vi "4080_display_source.vi"(0 "Module Address":u8) -> ()   [LabVIEW 2010]
panel:
  in  "Port Name":string="MainNetwork"
  in  "Data Source":u16(ring) items=["Counter0", "Counter1", "Host"]
  out "Read":string=">+00.000"
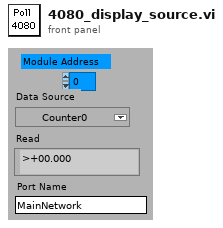
[diagram p1: front panel]
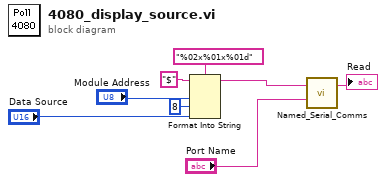
[diagram p0: block diagram]
diagram:
  n1 = Format Into String(format string="%02x%01x%01d", initial string="$", "Module Address", u8 8 ("Channel"), "Data Source") -> (resulting string=w1:string)  [unwired: 1 in, 1 out]
  n2 = call "Named_Serial_Comms.vi"("Write String"=w1, "Port Name"="Port Name") -> ("Read"=→"Read":string)  [unwired: 10 in, 3 out]
